vi "LabviewDemo.vi"() -> ()   [LabVIEW 2021]
uses:
  vmmsolib/vmmsolib.lvlib
panel:
  out "Support Samples":u32[](array[numeric])
  out "InitDll Return":i32
  out "Device is OK?":i32
  out "FinishDll Return":i32
  out "Voltage Wave":dbl[](graph)
  out "Voltage Array":dbl[](array[numeric]) caption="采集电压数组"
  out "ReadVoltageData Return":u32
  in  "Stop":bool
  out "Capture Return":i32
  out "Sample Success？":i32
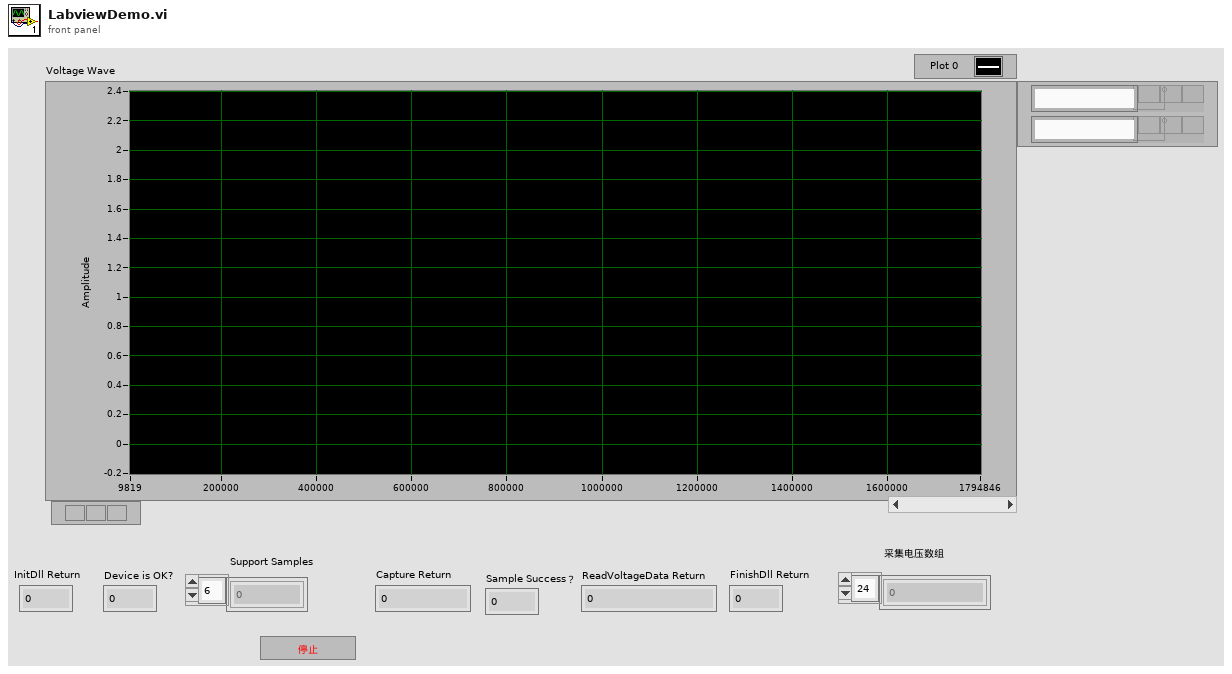
[diagram p1: front panel]
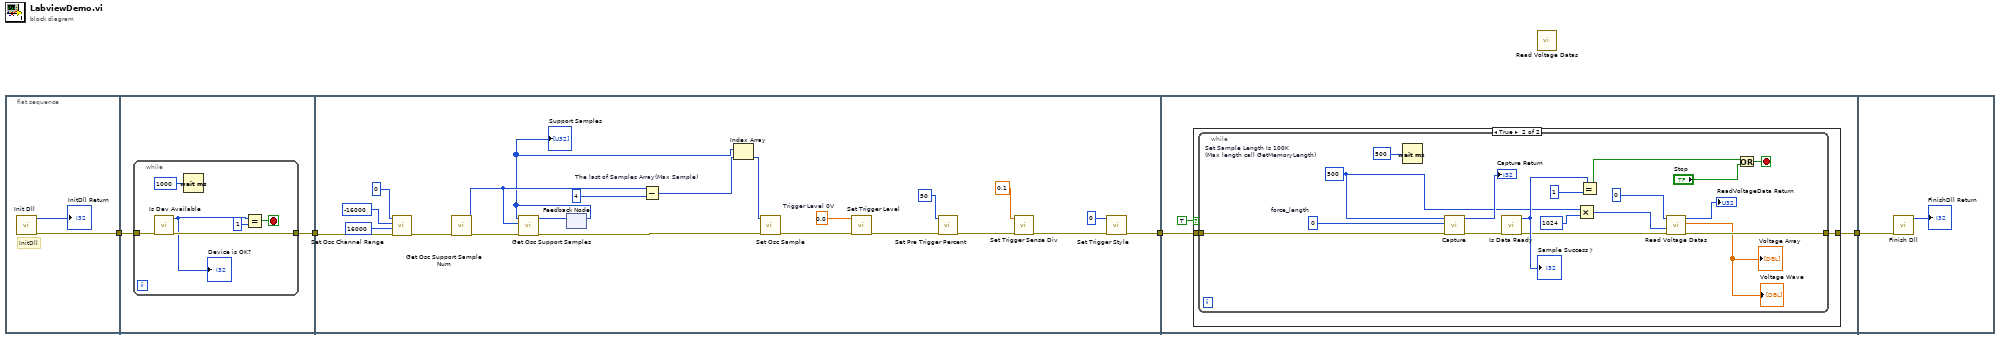
[diagram p0: block diagram]
diagram:
  n1 = flat-sequence {
    tunnel: [w6] -> w4
    tunnel: w4 -> [w8]
    tunnel: [w7] -> w3
    tunnel: w3 -> [w34]
    tunnel: [w26] -> w2
    tunnel: w2 -> [w39]
    tunnel: [w37] -> w1
    tunnel: w1 -> [w61]
    frame #0 {
      # "InitDll"
      n2 = call "Init Dll.vi"() -> ("error out"=w6:errorcluster, "function return"=→"InitDll Return":i32)  [unwired: 10 in]
    }
    frame #1 {
      n3 = while {
        tunnel: w8 -> [w11]
        tunnel: [w10] -> w7
        stop <- w12 stop-if-true
        n4 = call "Is Dev Available.vi"("error in (no error)"=w11) -> ("error out"=w10:errorcluster, "function return"=w9:i32)  [unwired: 9 in]
        "Device is OK?" <- w9
        n5 = Wait (ms)(milliseconds to wait=u32 1000 ("等待时间（毫秒）")) -> ()  [unwired: 1 out]
        n6 = Equal?(x=w9, y=1) -> (x = y?=w12:bool)
      }
    }
    frame #2 {
      w24 = sgl 0.0  # Trigger Level 0V
      n7 = call "Set Osc Channel Range.vi"("error in (no error)"=w34, "maxmv"=16000 ("minmv"), "minmv"=-16000, "channel"=0) -> ("error out"=w23:errorcluster)  [unwired: 6 in, 1 out]
      n8 = call "Get Osc Support Sample Num.vi"("error in (no error)"=w23) -> ("error out"=w22:errorcluster, "function return"=w17:i32)  [unwired: 9 in]
      n9 = feedback #1() -> (w15:u32[])  [unwired: 1 in]
      "Support Samples" <- w15
      n10 = call "Get Osc Support Samples.vi"("error in (no error)"=w22, "maxnum"=w17, "sample"=w15) -> ("error out"=w21:errorcluster, "sample out"=w16:u32[])  [unwired: 6 in, 1 out]
      n11 = feedback-in #1(w16) -> ()
      n12 = Subtract "The last of Samples Array(Max Sample)"(x=w17, y=4 ("front")) -> (x-y=w19:i32)
      n13 = Index Array(array=w15, index=w19) -> (element=w20:u32)
      n14 = call "Set Osc Sample.vi"("error in (no error)"=w21, "sample"=w20) -> ("error out"=w31:errorcluster)  [unwired: 8 in, 1 out]
      n15 = call "Set Trigger Level.vi"("error in (no error)"=w31, "level"=w24) -> ("error out"=w29:errorcluster)  [unwired: 9 in]
      n16 = call "Set Pre Trigger Percent.vi"("error in (no error)"=w29, "front"=50) -> ("error out"=w28:errorcluster)  [unwired: 9 in]
      n17 = call "Set Trigger Sense Div.vi"("error in (no error)"=w28, "sense"=0.1) -> ("error out"=w27:errorcluster)  [unwired: 9 in]
      n18 = call "Set Trigger Style.vi"("error in (no error)"=w27, "style"=u32 0) -> ("error out"=w26:errorcluster)  [unwired: 9 in]
    }
    frame #3 {
      n19 = case shown="True" TRUE {
        tunnel: w39 -> [_ w40]
        tunnel: [_ w41] -> w37
        frame False {
        }
        frame True {
          n20 = while {
            tunnel: [w48] -> w41
            tunnel: w40 -> [w52]
            stop <- w56 stop-if-true
            w45 = u32 500  # Set Sample Length Is 100K (Max length call GetMemoryLength)
            w50 = i8 0  # force_length
            n21 = Wait (ms)(milliseconds to wait=u32 500 ("等待时间（毫秒）")) -> ()  [unwired: 1 out]
            n22 = call "Capture.vi"("error in (no error)"=w52, "capture_channel"=w50, "length"=w45) -> ("error out"=w51:errorcluster, "function return"=→"Capture Return":i32)  [unwired: 7 in]
            n23 = call "Is Data Ready.vi"("error in (no error)"=w51) -> ("error out"=w49:errorcluster, "function return"=w55:i32)  [unwired: 9 in]
            "Sample Success？" <- w55
            n24 = Multiply(x=w45, y=1024) -> (x*y=w44:u32)
            n25 = Equal?(x=w55, y=1) -> (x = y?=w53:bool)
            n26 = call "Read Voltage Datas.vi"("error in (no error)"=w49, "length"=w44, "channel"=i8 0) -> ("error out"=w48:errorcluster, "buffer out"=→"Voltage Array" →"Voltage Wave":dbl[], "function return"=→"ReadVoltageData Return":u32)  [unwired: 6 in]
            n27 = Or(x=w53, y="Stop") -> (x .or. y?=w56:bool)
          }
        }
      }
    }
    frame #4 {
      n28 = call "Finish Dll.vi"("error in (no error)"=w61) -> ("function return"=→"FinishDll Return":i32)  [unwired: 9 in, 1 out]
    }
  }
  n29 = call "Read Voltage Datas.vi"() -> ()  [unwired: 9 in, 3 out]
